vi "GEA3 String Remove All Spaces.vi"(0 "Input String":string, 11 "error in (no error)":errorcluster) -> (4 "Spaces Removed":string, 15 "error out":errorcluster)   [LabVIEW 2016]
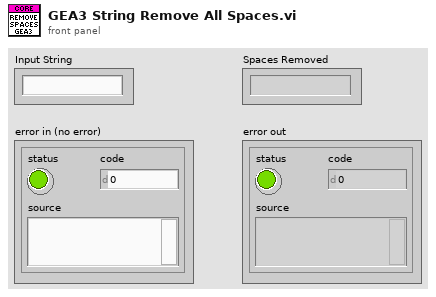
[diagram p1: front panel]
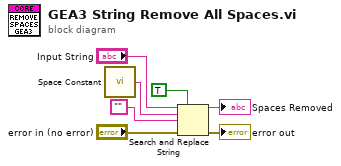
[diagram p0: block diagram]
diagram:
  n1 = call <vilib>:"Space Constant.vi"() -> ("String"=w5:string)
  n2 = Search and Replace String(replace all?=TRUE ("replace all? (F)"), input string="Input String", search string=w5, replace string="", error in="error in (no error)") -> (result string=→"Spaces Removed":string, error out=→"error out":errorcluster)  [unwired: 3 in, 2 out]
